vi "Calculate Incoming Protections.vi"(7 "Frame Count":i32, 8 "error in (no error)":errorcluster, 10 "Signal Settings":T1 {"Protection Configuration"."CRC Channels"."Data Type" items=["Signed", "Unsigned", "IEEE Float"]}) -> ()   [LabVIEW 2015, in "Protection and Counter Support Engine.lvlib"]
uses:
  Protection and Counter Support Engine.lvlib
  <vilib>/xnet/xnet.llb/XNET Convert (Signal to Frame Raw).vi
  Shared/Types/Exported Counter Settings.ctl
  Shared/Protection and Counter Support Shared.lvlib
  Shared/Types/XNET Signal Configuration.ctl
  Shared/Types/Protection Type.ctl
  Shared/Types/Exported Protection Settings.ctl
  Shared/Types/Exported Signal Settings.ctl
panel:
  out "Calculation Value":u8
  out "Previous Signal Values Out":dbl[](array[numeric])
  in  "Previous Signal Values In":dbl[](array[numeric])
  out "error out":errorcluster
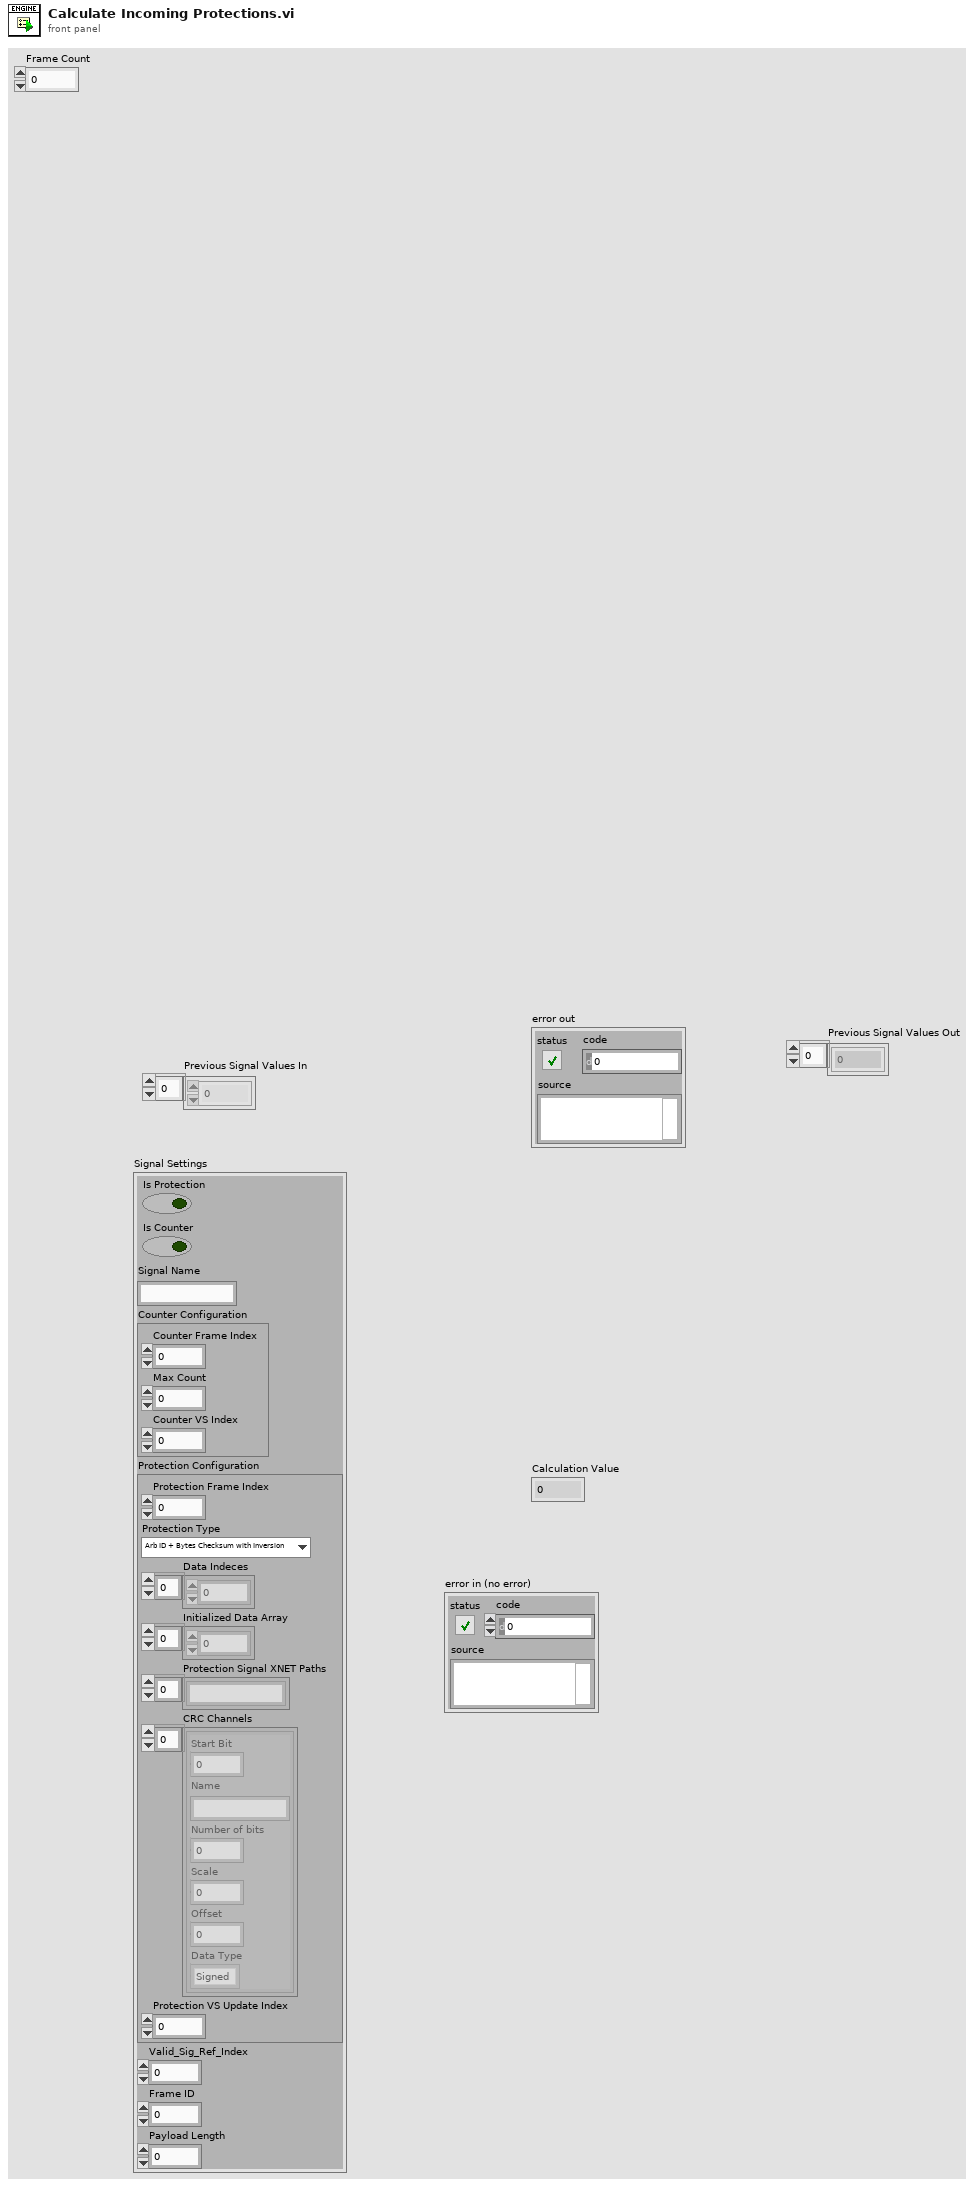
[diagram p1: front panel]
types:
  T1 = typedef "Protection and Counter Support Shared.lvlib/Exported Signal Settings.ctl" = cluster{"Is Protection":bool, "Is Counter":bool, "Signal Name":string, "Counter Configuration":T2, "Protection Configuration":T3, "Valid_Sig_Ref_Index":i32, "Frame ID":u32, "Payload Length":u32}
  T2 = typedef "Protection and Counter Support Shared.lvlib/Exported Counter Settings.ctl" = cluster{"Counter Frame Index":i32, "Max Count":dbl, "Counter VS Index":i32}
  T3 = typedef "Protection and Counter Support Shared.lvlib/Exported Protection Settings.ctl" = cluster{"Protection Frame Index":i32, "Protection Type":T4, "Data Indeces":i32[], "Initialized Data Array":dbl[], "Protection Signal XNET Paths":string[], "CRC Channels":T5[], "Protection VS Update Index":i32}
  T4 = typedef "Protection and Counter Support Shared.lvlib/Protection Type.ctl" = enum16{"Arb ID + Bytes Checksum with Inversion", "Arb ID + Bytes CRC with Inversion", "Reversed Raw Signal Checksum with Inversion"}
  T5 = typedef "Protection and Counter Support Shared.lvlib/XNET Signal Configuration.ctl" = cluster{"Start Bit":i32, "Name":string, "Number of bits":i32, "Scale":dbl, "Offset":dbl, "Data Type":u32}
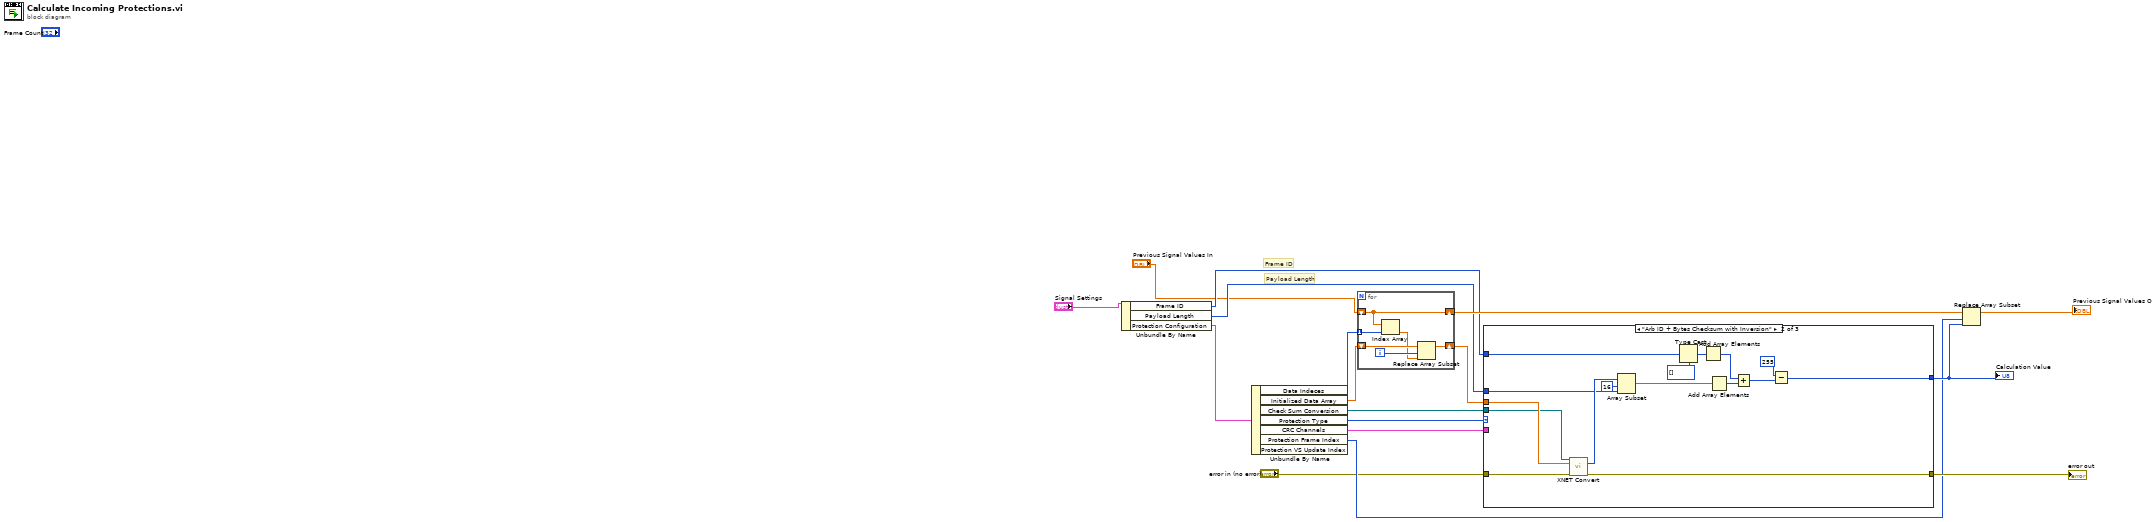
[diagram p0: block diagram]
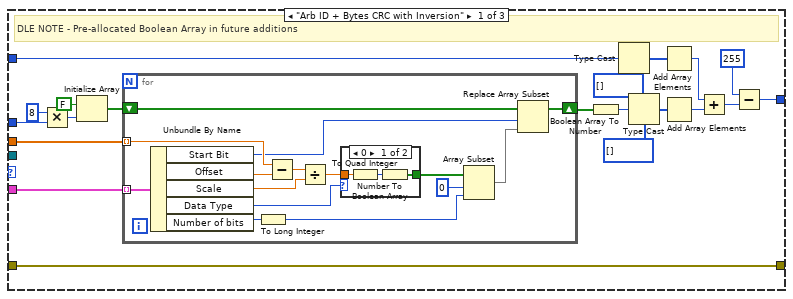
[diagram p2: hidden frame]
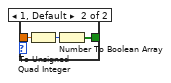
[diagram p3: hidden frame]
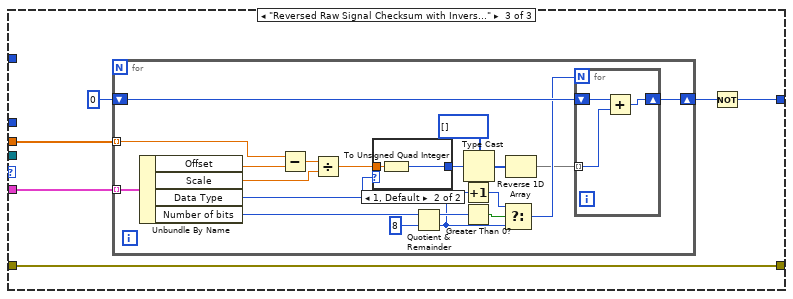
[diagram p4: hidden frame]
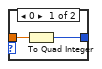
[diagram p5: hidden frame]
diagram:
  # "Payload Length"
  # "Frame ID"
  n1 = Unbundle By Name("Signal Settings") -> ("Frame ID"=w5:u32, "Payload Length"=w4:u32, "Protection Configuration"=w6:T3)
  n2 = Unbundle By Name(w6) -> ("Data Indeces"=w16:i32[], "Initialized Data Array"=w14:dbl[], "Check Sum Conversion"=w8:refnum<k21>, "Protection Type"=w9:T4, "CRC Channels"=w17:T5[], "Protection Frame Index"=w7:i32, "Protection VS Update Index"=w10:i32)
  n3 = for {
    shift-right: [w23] -> w15
    shift-left: "Previous Signal Values In" -> [w23]
    tunnel: w16 -> [w24] mode=indexing
    shift-right: [w19] -> w13
    shift-left: w14 -> [w22]
    i -> [w21]
    n4 = Index Array(array=w23, index=w24) -> (element=w20:dbl)
    n5 = Replace Array Subset(array=w22, new element=w20, index=w21) -> (w19:dbl[])
  }
  n6 = case shown="\"Arb ID + Bytes Checksum with Inversion\"" w9 {
    tunnel: w5 -> [w42 w79 _]
    tunnel: [w37 w74 w83] -> w11
    tunnel: "error in (no error)" -> [w33 w73 w82]
    tunnel: [w33 w72 w82] -> w12
    tunnel: w17 -> [w31 _ w85]
    tunnel: w13 -> [w32 w69 w84]
    tunnel: w8 -> [_ w68 _]
    tunnel: w4 -> [w27 w67 _]
    frame "Arb ID + Bytes CRC with Inversion" {
      # "DLE NOTE - Pre-allocated Boolean Array in future additions"
      n7 = Multiply(x=u32 8, y=w27) -> (x*y=w28:u32)
      n8 = Initialize Array(FALSE, w28) -> (w30:bool[])
      n9 = for {
        tunnel: w31 -> [w59] mode=indexing
        shift-right: [w50] -> w36
        shift-left: w30 -> [w52]
        tunnel: w32 -> [w49] mode=indexing
        n10 = Unbundle By Name(w59) -> ("Start Bit"=w46:i32, "Offset"=w58:dbl, "Scale"=w56:dbl, "Data Type"=w48:u32, "Number of bits"=w54:i32)
        n11 = To Long Integer(number=w54) -> (32bit integer=w45:i32)
        n12 = Subtract(x=w49, y=w58) -> (x-y=w57:dbl)
        n13 = Divide(x=w57, y=w56) -> (x/y=w55:dbl)
        n14 = case shown="0" w48 {
          tunnel: w55 -> [w62 w65]
          tunnel: [w60 w63] -> w47
          frame 0 {
            n15 = To Quad Integer(1:w62) -> (0:w61:i64)
            n16 = Number To Boolean Array(number=w61) -> (Boolean array=w60:bool[])
          }
          frame 1, Default {
            n17 = To Unsigned Quad Integer(1:w65) -> (0:w64:u64)
            n18 = Number To Boolean Array(number=w64) -> (Boolean array=w63:bool[])
          }
        }
        n19 = Array Subset(array=w47, index=0, length=w45) -> (w51:bool[])
        n20 = Replace Array Subset(array=w52, new element=w51, index=w46) -> (w50:bool[])
      }
      n21 = Boolean Array To Number(Boolean array=w36) -> (number=w35:u64)
      n22 = Type Cast(type=u8[] [], x=w42) -> (*(type *) &x=w41:u8[])
      n23 = Type Cast(type=u8[] [], x=w35) -> (*(type *) &x=w25:u8[])
      n24 = Add Array Elements(numeric array=w41) -> (sum=w40:u8)
      n25 = Add Array Elements(numeric array=w25) -> (sum=w44:u8)
      n26 = Add(x=w40, y=w44) -> (x+y=w39:u8)
      n27 = Subtract(x=u8 255, y=w39) -> (x-y=w37:u8)
    }
    frame "Arb ID + Bytes Checksum with Inversion" {
      n28 = call-poly <vilib>:"XNET Convert.vi"("session in"=w68, "signal data"=w69, "error in (no error)"=w73) -> ("frame data"=w70:u8[], "error out"=w72:errorcluster)  [unwired: 10 in, 1 out]
      n29 = Array Subset(array=w70, index=16 ("length"), length=w67) -> (w66:u8[])
      n30 = Type Cast(type=u8[] [], x=w79) -> (*(type *) &x=w78:u8[])
      n31 = Add Array Elements(numeric array=w78) -> (sum=w77:u8)
      n32 = Add Array Elements(numeric array=w66) -> (sum=w81:u8)
      n33 = Add(x=w77, y=w81) -> (x+y=w76:u8)
      n34 = Subtract(x=u8 255, y=w76) -> (x-y=w74:u8)
    }
    frame "Reversed Raw Signal Checksum with Inversion" {
      n35 = for {
        tunnel: w85 -> [w107] mode=indexing
        tunnel: w84 -> [w104] mode=indexing
        shift-right: [w101] -> w86
        shift-left: u8 0 -> [w102]
        n36 = Unbundle By Name(w107) -> ("Offset"=w106:dbl, "Scale"=w105:dbl, "Data Type"=w103:u32, "Number of bits"=w99:i32)
        n37 = Subtract(x=w104, y=w106) -> (x-y=w98:dbl)
        n38 = Divide(x=w98, y=w105) -> (x/y=w97:dbl)
        n39 = case shown="1, Default" w103 {
          tunnel: w97 -> [w112 w114]
          tunnel: [w111 w113] -> w100
          frame 0 {
            n40 = To Quad Integer(1:w112) -> (0:w111:i64)
          }
          frame 1, Default {
            n41 = To Unsigned Quad Integer(1:w114) -> (0:w113:u64)
          }
        }
        n42 = Quotient & Remainder(x=w99, y=8) -> (x-y*floor(x/y)=w94:i32, floor(x/y)=w92:i32)
        n43 = Increment(x=w92) -> (x+1=w93:i32)
        n44 = Greater Than 0?(x=w94) -> (x > 0?=w95:bool)
        n45 = Type Cast(type=u8[] [], x=w100) -> (*(type *) &x=w89:u8[])
        n46 = Select(t=w93, s=w95, f=w92) -> (s? t:f=w91:i32)
        n47 = Reverse 1D Array(array=w89) -> (reversed array=w88:u8[])
        n48 = for {
          N: w91 -> [_]
          tunnel: w88 -> [w109] mode=indexing
          shift-right: [w108] -> w101
          shift-left: w102 -> [w110]
          n49 = Add(x=w110, y=w109) -> (x+y=w108:u8)
        }
      }
      n50 = Not(x=w86) -> (.not. x?=w83:u8)
    }
  }
  "error out" <- w12
  "Calculation Value" <- w11
  n51 = Replace Array Subset(array=w15, new element=w11, index=w7) -> (→"Previous Signal Values Out":dbl[])
